vi "json To Minimized String - array path.vi"(7 "pretty print?":bool, 8 "error in (no error)":errorcluster, 10 "path":string[](array[string]), 11 "JSON Document in":refnum<class "JSON Document.lvclass">) -> (0 "error out":errorcluster, 2 "json string":string, 3 "JSON Document out":refnum<class "JSON Document.lvclass">)   [LabVIEW 2015, in "JSON Document.lvclass"]
uses:
  JSON Document.lvclass
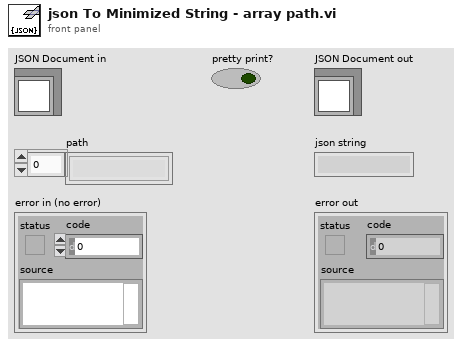
[diagram p1: front panel]
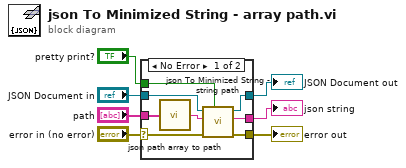
[diagram p0: block diagram]
diagram:
  n1 = case shown="No Error" "error in (no error)" {
    selector: "error in (no error)" -> [w11 w17]
    tunnel: [w12 w17] -> w6
    tunnel: [w14 w16] -> w4
    tunnel: "JSON Document in" -> [w15 w16]
    tunnel: [w13 _] -> w3
    tunnel: "path" -> [w9 _]
    tunnel: "pretty print?" -> [w8 _]
    frame No Error {
      n2 = call "json path array to path.vi"("path"=w9) -> ("String"=w10:string)
      n3 = call "json To Minimized String - string path.vi"("pretty print?"=w8, "error in (no error)"=w11, "path"=w10, "JSON Document in"=w15) -> ("error out"=w12:errorcluster, "json string"=w13:string, "JSON Document out"=w14:refnum<class "JSON Document.lvclass">)  [unwired: 5 in]
    }
    frame Error {
    }
  }
  "error out" <- w6
  "JSON Document out" <- w4
  "json string" <- w3
